vi "RPT Comaristion.vi"(10 "True":bool) -> (1 "Fail":bool)   [LabVIEW 2015]
uses:
  Galobal variable_TI.vi
  Project Setup/Globle Variable/GR_Servo.vi
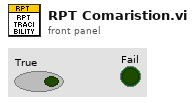
[diagram p1: front panel]
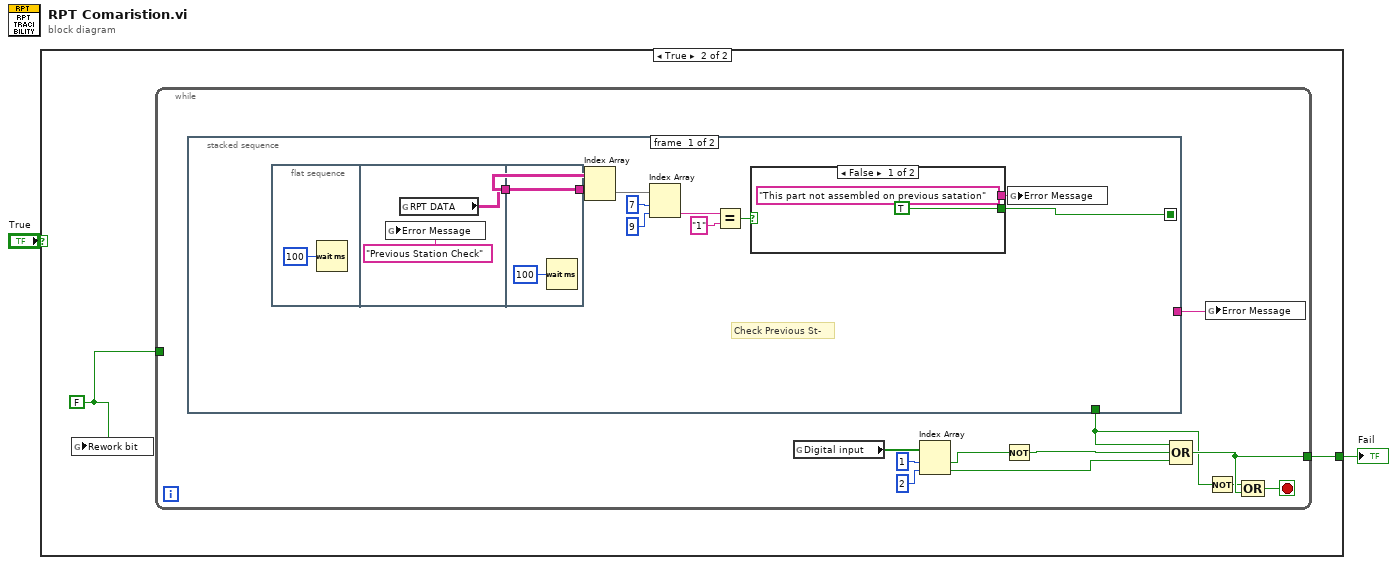
[diagram p0: block diagram]
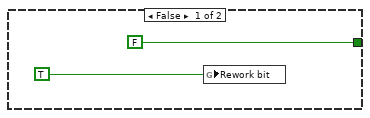
[diagram p2: hidden frame]
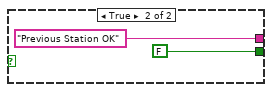
[diagram p3: hidden frame]
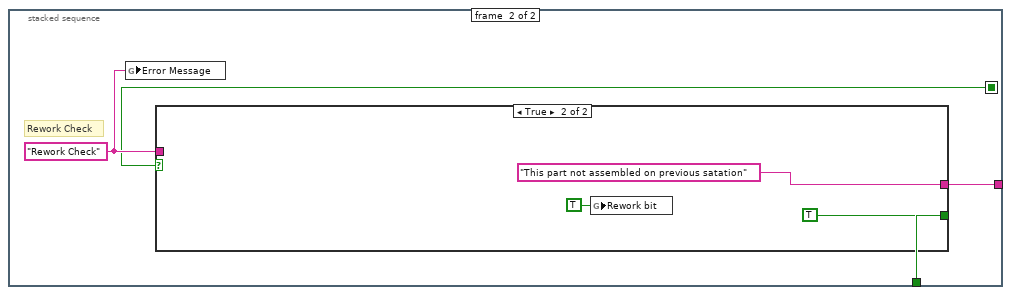
[diagram p4: hidden frame]
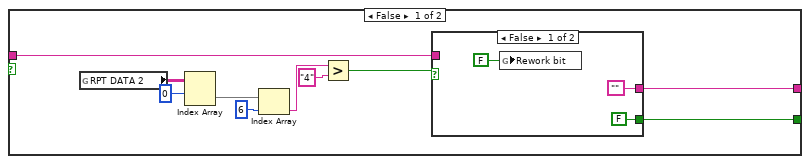
[diagram p5: hidden frame]
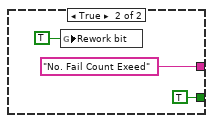
[diagram p6: hidden frame]
diagram:
  n1 = case shown="True" "True" {
    tunnel: [FALSE w6] -> w1
    frame False {
      n2 = global write "Galobal variable_TI.vi" "Rework bit"(TRUE ("Rework bit")) -> ()
    }
    frame True {
      w5 = FALSE ("Rework bit")
      n3 = global write "Galobal variable_TI.vi" "Rework bit"(w5) -> ()
      n4 = while {
        tunnel: [w10] -> w6
        tunnel: w5 -> [_]
        stop <- w11 stop-if-true
        n5 = stacked-sequence {
          seq-local: [w20 _] -> [_ w39]
          tunnel: [_ w38] -> w9
          tunnel: [_ w37] -> w8
          frame #0 {
            # "Check Previous St-"
            n6 = flat-sequence {
              tunnel: [w30] -> w18
              tunnel: [w32] -> w22
              tunnel: w18 -> [w32]
              frame #0 {
                n7 = Wait (ms)(milliseconds to wait=u32 100) -> ()  [unwired: 1 out]
              }
              frame #1 {
                n8 = global write "GR_Servo.vi" "Error Message"("Previous Station Check") -> ()
                n9 = global read "GR_Servo.vi" "RPT DATA"() -> (w30:string[][])
              }
              frame #2 {
                n10 = Wait (ms)(milliseconds to wait=u32 100) -> ()  [unwired: 1 out]
              }
            }
            n11 = Index Array(array=w22) -> (element=w24:string[])  [unwired: 2 in]
            n12 = Index Array(array=w24, index #1=7 ("index"), index #2=9 ("index")) -> (element #2=w27:string)  [unwired: 1 out]
            n13 = Equal?(x=w27, y="1") -> (x = y?=w19:bool)
            n14 = case shown="False" w19 {
              tunnel: ["This part not assembled on previous satation" "Previous Station OK"] -> w21
              tunnel: [TRUE FALSE] -> w20
              frame False {
              }
              frame True {
              }
            }
            n15 = global write "GR_Servo.vi" "Error Message"(w21) -> ()
          }
          frame #1 {
            w40 = "Rework Check"
            # "Rework Check"
            n16 = global write "GR_Servo.vi" "Error Message"(w40) -> ()
            n17 = case shown="True" w39 {
              tunnel: w40 -> [w45 _]
              tunnel: [w44 "This part not assembled on previous satation"] -> w38
              tunnel: [w43 TRUE] -> w37
              frame False {
                n18 = global read "GR_Servo.vi" "RPT DATA 2"() -> (w47:string[][])
                n19 = Index Array(array=w47, index (row)=0) -> (element=w50:string[])  [unwired: 1 in]
                n20 = Index Array(array=w50, index=6) -> (element=w46:string)
                n21 = Greater?(x=w46, y="4") -> (0:w41:bool)
                n22 = case shown="False" w41 {
                  tunnel: ["" "No. Fail Count Exeed"] -> w44
                  tunnel: w45 -> [_ _]
                  tunnel: [FALSE TRUE] -> w43
                  frame False {
                    n23 = global write "Galobal variable_TI.vi" "Rework bit"(FALSE) -> ()
                  }
                  frame True {
                    n24 = global write "Galobal variable_TI.vi" "Rework bit"(TRUE) -> ()
                  }
                }
              }
              frame True {
                n25 = global write "Galobal variable_TI.vi" "Rework bit"(TRUE ("Rework bit")) -> ()
              }
            }
          }
        }
        n26 = global read "Galobal variable_TI.vi" "Digital input"() -> (w17:bool[])
        n27 = Index Array(array=w17, index #1=1 ("index"), index #2=2 ("index")) -> (element #1=w14:bool, element #2=w12:bool)
        n28 = Not(x=w14) -> (.not. x?=w13:bool)
        n29 = Compound Arithmetic op=OR(w8, w13, w12) -> (w10:bool)
        n30 = global write "GR_Servo.vi" "Error Message"(w9) -> ()
        n31 = Not(x=w8) -> (.not. x?=w7:bool)
        n32 = Compound Arithmetic op=OR(w7, w10) -> (w11:bool)
      }
    }
  }
  "Fail" <- w1
